vi "Save Recall Waveforms.vi"(8 "error in (no error)":errorcluster, 10 "Waveforms Operation (0: Save)":u16(ring) items=["Save", "Recall"], 11 "VISA resource name":refnum<visa-resource-name>) -> (0 "error out":errorcluster, 3 "VISA resource name out":refnum<visa-resource-name>)   [LabVIEW 2018, in "Agilent PSG MXG Series.lvlib"]
doc: "(1) Stores from the internal BBG memory to the active media. (2) Loads all of the waveforms in the active media to the internal BBG memory. \nThe active media is either internal non-volatile memory storage media or an external storage media connected to the front-panel USB port.\n\n<b>Note:</b>\nThis VI is valid on N5172B that installs with <B>Option 653</B> or <B>Option 655</B>, or N5182B that installs with <B>Option 656</B> or <B>Option 657</B>, or N5162A, N5182A."
uses:
  Agilent PSG MXG Series.lvlib
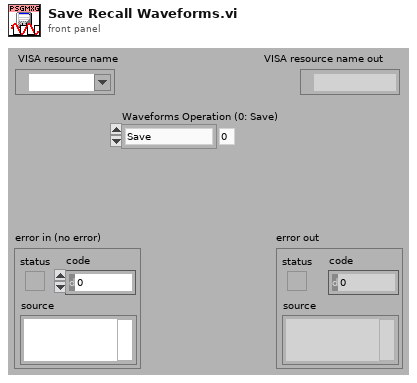
[diagram p1: front panel]
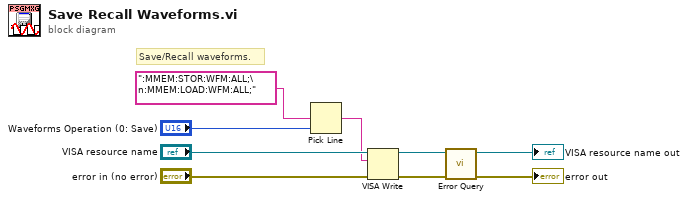
[diagram p0: block diagram]
diagram:
  # "Save/Recall waveforms."
  n1 = Pick Line(multi-line string=":MMEM:STOR:WFM:ALL;\n:MMEM:LOAD:WFM:ALL;", line index="Waveforms Operation (0: Save)") -> (output string=w3:string)  [unwired: 1 in]
  n2 = VISA Write(VISA resource name="VISA resource name", write buffer=w3, error in (no error)="error in (no error)") -> (VISA resource name out=w9:refnum<visa-resource-name>, error out=w8:errorcluster)  [unwired: 1 out]
  n3 = call "Error Query.vi"("error in (no error)"=w8, "VISA resource name"=w9) -> ("error out"=→"error out":errorcluster, "VISA resource name out"=→"VISA resource name out":refnum<visa-resource-name>)  [unwired: 8 out]
